vi "DHT12.vi"() -> ()   [LabVIEW 2020]
uses:
  lv_i2c_ad2/AD2 I2C/AD2 I2C.lvclass
  C:/Users/user/Documents/LabVIEW Data/lv_i2c_hal/I2C/I2C.lvclass
  lv_waveforms_toolkit/lv_waveforms_toolkit.lvlib
  lv_dht12/lv_dht12.lvlib
panel:
  out "Humidity":dbl
  out "Temperature":dbl
  in  "stop":bool
  out "Error Out":errorcluster
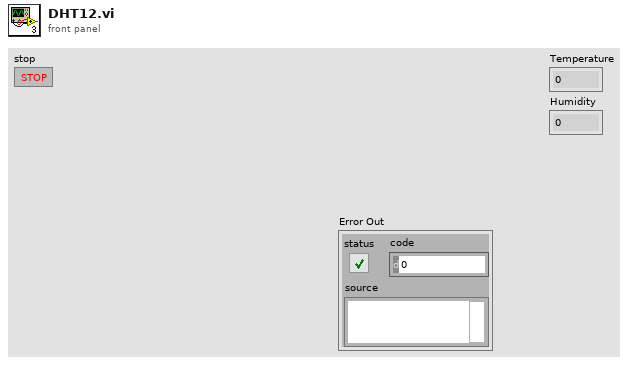
[diagram p1: front panel]
types:
  T1 = typedef "lv_waveforms_toolkit.lvlib/WFT Session.ctl" = cluster{"phdwf":i32, "Analog IO Configured":bool}
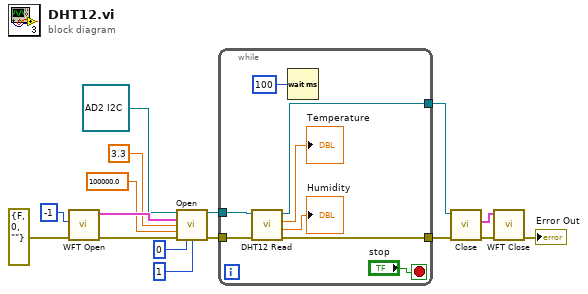
[diagram p0: block diagram]
diagram:
  n1 = call "WFT Open.vi"("Error In"=errorcluster {"status"=FALSE, "code"=0, "source"=""}, "idxDevice"=-1) -> ("Error Out"=w12:errorcluster, "WaveForms Session Out"=w13:T1)  [unwired: 7 in, 1 out]
  n2 = call "Open.vi"("AD2 I2C In"=refnum<class "AD2 I2C.lvclass"> refnum, "WaveForms Session In"=w13, "Power Supply Voltage"=3.3, "hz"=100000.0, "Error In"=w12, "SCL idxChannel"=0, "SDA idxChannel"=1) -> ("AD2 I2C Out"=w8:refnum<class "AD2 I2C.lvclass">, "Error Out"=w7:errorcluster)  [unwired: 7 in]
  n3 = while {
    tunnel: w8 -> [w24]
    tunnel: w7 -> [w23]
    tunnel: [w21] -> w6
    tunnel: [w20] -> w5
    stop <- "stop" stop-if-true
    n4 = call "DHT12 Read.vi"("Error In"=w23, "I2C In"=w24) -> ("Error Out"=w21:errorcluster, "Humidity"=→"Humidity":dbl, "Temperature"=→"Temperature":dbl, "I2C Out"=w20:refnum<class "AD2 I2C.lvclass">)  [unwired: 5 in, 1 out]
    n5 = Wait (ms)(milliseconds to wait=u32 100) -> ()  [unwired: 1 out]
  }
  n6 = call "Close.vi"("Error In"=w6, "AD2 I2C In"=w5) -> ("Error Out"=w10:errorcluster, "WaveForms Session Out"=w9:T1)  [unwired: 7 in, 1 out]
  n7 = call "WFT Close.vi"("Error In"=w10, "WaveForms Session In"=w9) -> ("Error Out"=→"Error Out":errorcluster)  [unwired: 8 in, 1 out]
